vi "MasterDirectory.vi"() -> (0 "Master Directory":path=path "C:/CuspControl")   [LabVIEW 2018]
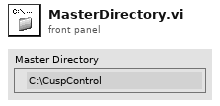
[diagram p1: front panel]
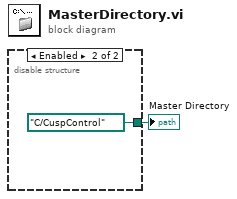
[diagram p0: block diagram]
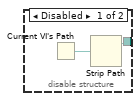
[diagram p2: hidden frame]
diagram:
  n1 = disable-structure shown="Enabled" {
    disable-tunnel: [w2 path "C:/CuspControl" ("Master Directory")] -> w1
    frame Disabled {
      n2 = Current VI's Path() -> (path=w3:path)
      n3 = Strip Path(path=w3) -> (stripped path=w2:path)  [unwired: 1 out]
    }
    frame Enabled {
    }
  }
  "Master Directory" <- w1
